vi "Find Ocean Optics.vi"(8 "Error In":errorcluster) -> (0 "Error Out":errorcluster, 3 "Devices":refnum<visa-resource-name>[](array[refnum]))   [LabVIEW 2016]
uses:
  <vilib>/Instr/_visa.llb/VISA Find Search Mode.ctl
  <vilib>/Utility/error.llb/Error Cluster From Error Code.vi
  <vilib>/ErrorRing/Error Ring.xnode
  <instrlib>/Ocean Optics 2000 4000/Ocean Optics 2000 4000.lvlib
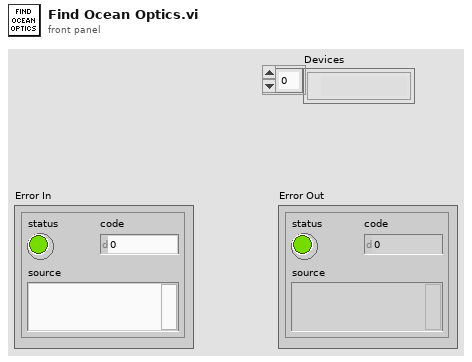
[diagram p1: front panel]
types:
  T1 = typedef "VISA Find Search Mode.ctl" = u32
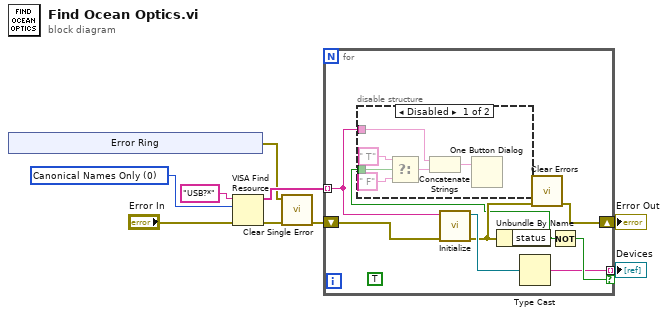
[diagram p0: block diagram]
diagram:
  w9 = T1 0 items=["Canonical Names Only"=0, "Aliases Only"=2, "Include Matching Aliases"=3, "Include All Aliases"=4] ("Search Mode")
  n1 = xnode "Error Ring"() -> ("error out"=w4:errorcluster)
  n2 = VISA Find Resource(8:"Error In", 10:w9, 11:"USB?*" ("expression (\"?*\")")) -> (0:w3:errorcluster, 3:w8:string[])  [unwired: 1 out]
  n3 = call "Clear Single Error.vi"("Error In"=w3, "Error to clear"=w4) -> ("Error Out"=w2:errorcluster)  [unwired: 8 in, 1 out]
  n4 = for {
    tunnel: w8 -> [w11] mode=indexing
    tunnel: [w14] -> w1 mode=indexing if=w16
    shift-right: [w12] -> w6
    shift-left: w2 -> [w17]
    (unwired) TRUE
    n5 = call <instrlib>:"Initialize.vi"("error in (no error)"=w17, "VISA resource name"=w11) -> ("error out"=w13:errorcluster, "VISA resource name out"=w15:refnum<visa-resource-name>)  [unwired: 8 in]
    n6 = Unbundle By Name(w13) -> ("status"=w10:bool)
    n7 = disable-structure shown="Disabled" {
      disable-tunnel: w10 -> [w22 _]
      disable-tunnel: w11 -> [w18 _]
      frame Disabled {
        n8 = Select(t=" T" ("concatenated string"), s=w22, f=" F" ("concatenated string")) -> (s? t:f=w19:string)
        n9 = Concatenate Strings(w18, w19) -> (w23:string)
        n10 = One Button Dialog(message=w23) -> ()  [unwired: 1 in, 1 out]
      }
      frame Enabled {
      }
    }
    n11 = Type Cast(x=w15) -> (*(type *) &x=w14:string)  [unwired: 1 in]
    n12 = call <vilib>:"Clear Errors.vi"("error in (no error)"=w13) -> ("error out"=w12:errorcluster)  [unwired: 5 in, 1 out]
    n13 = Not(x=w10) -> (.not. x?=w16:bool)
  }
  "Devices" <- w1
  "Error Out" <- w6
